vi "IDE_UART_Example.vi"() -> ()   [LabVIEW 2020]
uses:
  Subs/ColorText/Code.xctl
  Subs/Console XCtrl/Console_Xctrl.xctl
  Subs/Server XCtrl/Server.xctl
panel:
  in  "Files 2":bool
  in  "Open Server 2":bool
  in  "Help 2":bool
  in  "Name 2":string="code.py"
  in  "Save 2":bool
  in  "Stop 2":bool
  in  "Pyboard":string(xcontrol)="# UART Control\n#\n# This example shows how to use the serial port on your OpenMV Cam.   P4 (Tx), P5(Rx)\n\nimport utime\nfrom pyb import UART\n\nuart = UART(3, 115200)\n\nwhile(True):\n    if uart.any():\n        uart.read(uart.any())\n    uart.write(\"OpenMV\\r\")\n    utime.sleep(2)\n    \n    \n    "
  in  "Run 2":bool
  in  "Clean 2":bool
  in  "PC Save 2":bool
  in  "PC path 2":path
  in  "Clear 2":bool
  out "REPL 2":string(xcontrol)="\n>>> import time\n>>> from pyb import UART\n>>> uart = UART(3, 19200)\n>>> while(True):\n...     uart.write(\"Hello World!\\r\")\n...     time.sleep(1000)\n...     \n...     \n... \n13\n13\n13\n13\n13\nTraceback (most recent call last):\n  File \"<stdin>\", line 3, in <module>\nKeyboardInterrupt: \n>>> uart.write(\"Hello World!\\r\")\n13\n>>> uart = UART(3, 115200)\n>>> uart.write(\"Hello World!\\r\")\n13\n>>> time.sleep(1)\n>>> time.sleep(1000)\n>>> import utime\n>>> utime.sleep(1)\n>>> import utime\n>>> from pyb import UART\n>>> uart = UART(3, 115200)\n>>> while(True):\n...     if uart.any():\n...         uart.read(uart.any())\n...     uart.write(\"Hello World!\\r\")\n...     utime.sleep(2)\n...     \n...     \n... \n13\n13\n13\nTraceback (most recent call last):\n  File \"<stdin>\", line 5, in <module>\nKeyboardInterrupt: \n>>> import utime\n>>> from pyb import UART\n>>> uart = UART(3, 115200)\n>>> while(True):\n...     if uart.any():\n...         uart.read(uart.any())\n...     uart.write(\"OpenMV\\r\")\n...     utime.sleep(2)\n...     \n...     \n... \n7\nb'SPIKE\\r'\n7\nb'SPIKE\\r'\n7\nb'SPIKE\\r'\n7\nb'SPIKE\\r'\n7\nTraceback (most recent call last):\n  File \"<stdin>\", line 5, in <module>\nKeyboardInterrupt: \n>>> uart.\n__class__       __next__        any             read\nreadinto        readline        write           init\nCTS             IRQ_RXIDLE      RTS             deinit\nirq             readchar        sendbreak       writechar\n>>> uart"
  in  "Server 2":path(xcontrol)=path "/Users/crogers/GitHub/Summer2020/LabVIEWCode/Servers/Damien.vi"
  in  "Clean":bool
  in  "PC Save":bool
  in  "PC path":path
  in  "Files":bool
  in  "Open Server":bool
  in  "Help":bool
  in  "Server":path(xcontrol)=path "/Users/crogers/GitHub/Summer2020/LabVIEWCode/Servers/Jens.vi"
  out "REPL":string(xcontrol)="0], \"\", 0]}{\"m\":0,\"p\":[[0, []], [0, []], [0, []], [0, []], [0, []], [0, []], [-18, -2, 994], [3, 5, 1], [24, 1, 0], \"\", 0]}{\"m\":0,\"p\":[[0, []], [0, []], [0, []], [0, []], [0, []], [0, []], [-19, -3, 994], [3, 6, 1], [24, 1, 0], \"\", 0]}{\"m\":0,\"p\":[[0, []], [0, []], [0, []], [0, []], [0, []], [0, []], [-20, 0, 994], [3, 5, 1], [24, 1, 0], \"\", 0]}Traceback (most recent call last):\n  File \"main.py\", line 8, in <module>\n  File \"lib/hub/flash/hub_runtime.py\", line 1, in start\nKeyboardInterrupt: \nMicroPython v1.11-1139-gf7407e5a0 on 2020-06-19; LEGO Technic Large Hub with STM32F413xx\nType \"help()\" for more information.\n>>> {\"m\":4,\"p\":\"tapped\"}{\"m\":4,\"p\":\"rightside\"}{\"m\":4,\"p\":\"front\"}{\"m\":4,\"p\":\"rightside\"}{\"m\":4,\"p\":\"front\"}{\"m\":4,\"p\":\"tapped\"}\n>>> \n>>> \n>>> {\"m\":4,\"p\":\"tapped\"}\n>>> import hub, utime\n>>> hub.port.B.mode(hub.port.MODE_FULL_DUPLEX)\n>>> utime.sleep(1)\n>>> hub.port.B.baud(115200)\n>>> hub.port.B.write(hello sir!.encode()) \nTraceback (most recent call last):\n  File \"<stdin>\", line 1\nSyntaxError: invalid syntax\n>>> hub.port.B.read(100)\nb''\n>>> \n>>> hub.port.B.write('hello sir!'.encode()) # to write\n10\n>>> hub.port.B.read(100)\nb'hello sir!'\n>>> hub.port.B.read(100)\nb'\\xe0\\xe0\\xe0\\xe0\\xe0\\xe0\\xe0\\xe0\\xe0\\xe0\\xe0\\xe0\\xe0\\xe0\\xe0\\xe0\\xe0\\xe0\\xe0\\xe0\\xe0\\xe0\\xe0\\xe0\\xe0\\xe0\\xe0\\xe0\\xe0\\xe0\\xe0\\xe0\\xe0\\xe0\\xe0\\xe0\\xe0\\xe0\\xe0\\xe0\\xe0\\xe0\\xe0\\xe0\\xe0\\xe0\\xe0\\xe0\\xe0\\xe0\\xe0\\xe0\\xe0\\xe0\\xe0\\xe0\\xe0\\xe0\\xe0\\xe0\\xe0\\xe0\\xe0\\xe0\\xe0\\xe0\\xe0\\xe0\\xe0\\xe0\\xe0\\xe0\\xe0\\xe0\\xe0\\xe0\\xe0\\xe0\\xe0\\xe0\\xe0\\xe0\\xe0\\xe0\\xe0\\xe0\\xe0\\xe0\\xe0\\xe0\\xe0\\xe0\\xe0\\xe0\\xe0\\xe0\\xe0\\xe0\\xe0\\xe0'\n>>> hub.port.B.read(100)\nb'\\xe0\\xe0\\xe0\\xe0\\xe0\\xe0\\xe0\\xe0\\xe0\\xe0\\xe0\\xe0\\xe0\\xe0\\xe0\\xe0\\xe0\\xe0\\xe0\\xe0\\xe0\\xe0\\xe0\\xe0'\n>>> hub.port.B.read(100)\nb''\n>>> hub.port.B.read(100)\nb'\\xe0\\xe0\\xe0\\xe0\\xe0\\xe0\\xe0\\xe0\\xe0\\xe0\\xe0\\xe0\\xe0\\xe0\\xe0\\xe0\\xe0\\xe0\\xe0\\xe0\\xe0\\xe0\\xe0\\xe0\\xe0'\n>>> hub.port.B.read(100)\nb''\n>>> hub.port.B.read(100)\nb'Hello World!\\r'\n>>> \n>>> uart = hub.port.B\n>>> uart.\n__class__       read            write           baud\ncallback        device          info            mode\nmotor           pwm\n>>> uart.read()\nTraceback (most recent call last):\n  File \"<stdin>\", line 1, in <module>\nTypeError: function takes 2 positional arguments but 1 were given\n>>> uart.read(1000)\nb'Hello World!\\rHello World!\\rHello World!\\r'\n>>> import hub, utime\n>>> uart = hub.port.B\n>>> uart.mode(hub.port.MODE_FULL_DUPLEX)\n>>> uart.baud(115200)\n>>> hub.port.B.write('hello sir!'.encode()) \n10\n>>> hub.port.B.read(100)\nb''\n>>> while(True):\n...     uart.read(100)\n...     uart.write(\"SPIKE\\r\")\n...     utime.sleep(2)\n...     \n...     \n... \nb''\n6\nb''\n6\nb'OpenMV\\r'\n6\nb'OpenMV\\r'\n6\nb'OpenMV\\r'\n6\nb'OpenMV\\r'\n6\nTraceback (most recent call last):\n  File \"<stdin>\", line 4, in <module>\nKeyboardInterrupt: \n>>> def gotit():\n...     print(\n>>> {\"m\":4,\"p\":\"tapped\"}"
  in  "Clear":bool
  in  "Save":bool
  in  "Stop":bool
  in  "Run":bool
  in  "Name":string="code.py"
  in  "SPIKE Prime":string(xcontrol)="import hub, utime\n\nuart = hub.port.B\nuart.mode(hub.port.MODE_FULL_DUPLEX)\nuart.baud(115200)\n\nwhile(True):\n    uart.read(100)\n    uart.write(\"SPIKE\\r\")\n    utime.sleep(2)\n    \n    \n    "
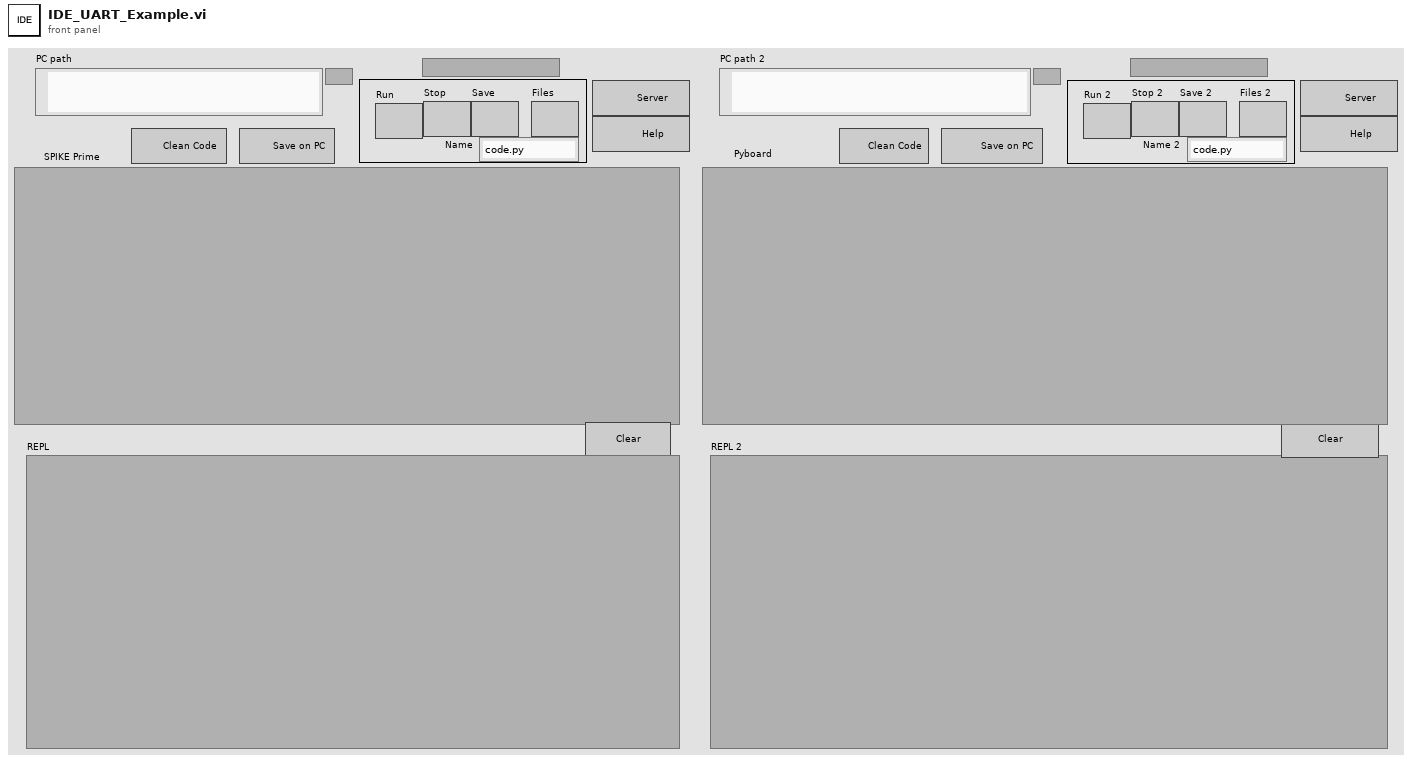
[diagram p1: front panel]
types:
  T1 = cluster{"Quote":u32, "Comment":u32, "Python":u32, "Text":u32, "Triple Quote":u32, "function":u32, "Line numbers":u32, "REPL Err":u32, "REPL Text":u32, "Text Bkgd":u32, "REPL Bkgd":u32}
  T2 = enum8{"Enabled", "Disabled", "Disabled and Grayed Out"}
  T3 = typedef "eventvkey.ctl" = enum16{"ASCII", "Enter", "Return", "Shift", "Ctrl", "Alt", "Cmd", "Opt", "Caps", "NumLock", "Clear", "Break", "Up", "Down", "Left", "Right", "Insert", "Delete", "Home", "End", "PageUp", "PageDown", "Escape", "Help", "Pause", "ScrollLock", "F1", "F2", "F3", "F4", "F5", "F6", "F7", "F8", "F9", "F10", "F11", "F12", "F13", "F14", "F15", "F16", "F17", "F18", "F19", "F20", "F21", "F22", "F23", "F24", "Play", "VolumeUp", "VolumeDown", "Mute", "Two Byte Char"}
  T4 = cluster{"Shift":bool, "Ctrl":bool, "Alt":bool, "Cmd":bool, "Opt":bool}
  T5 = cluster{"Char":i16, "VKey":T3, "PlatMods":cluster{"Shift":bool, "Ctrl":bool, "Alt":bool, "Cmd":bool, "Opt":bool}}
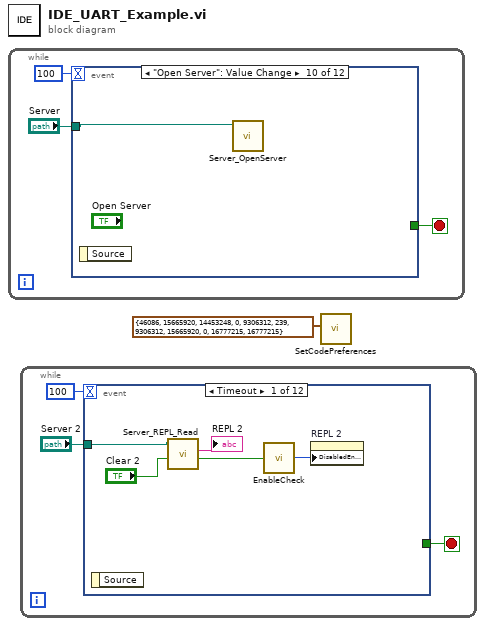
[diagram p0: block diagram]
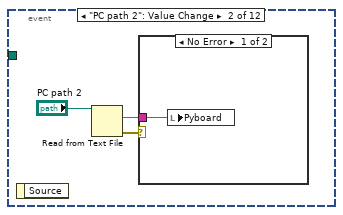
[diagram p2: hidden frame]
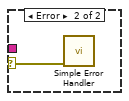
[diagram p3: hidden frame]
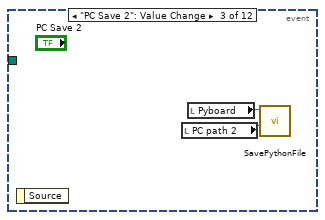
[diagram p4: hidden frame]
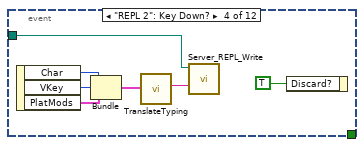
[diagram p5: hidden frame]
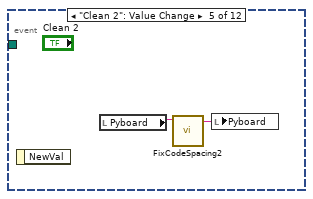
[diagram p6: hidden frame]
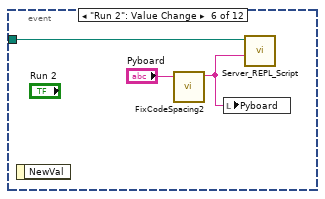
[diagram p7: hidden frame]
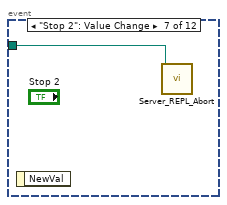
[diagram p8: hidden frame]
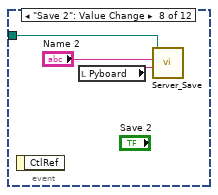
[diagram p9: hidden frame]
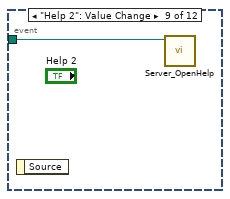
[diagram p10: hidden frame]
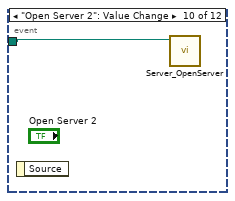
[diagram p11: hidden frame]
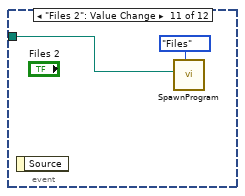
[diagram p12: hidden frame]
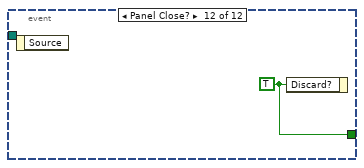
[diagram p13: hidden frame]
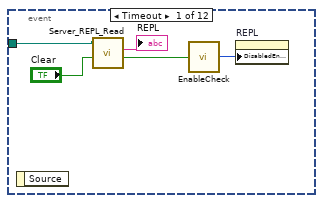
[diagram p14: hidden frame]
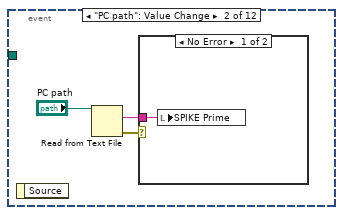
[diagram p15: hidden frame]
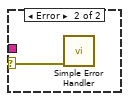
[diagram p16: hidden frame]
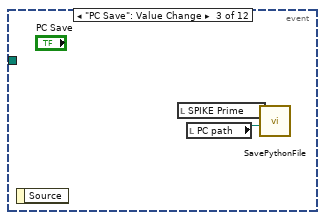
[diagram p17: hidden frame]
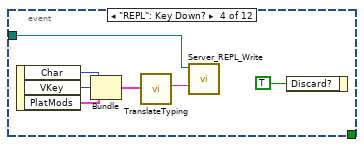
[diagram p18: hidden frame]
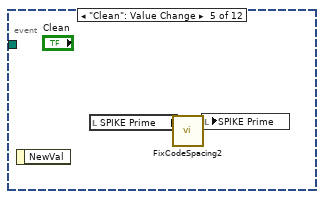
[diagram p19: hidden frame]
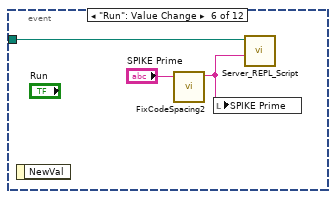
[diagram p20: hidden frame]
diagram:
  n1 = while {
    stop <- w3 stop-if-true
    n2 = event shown="[9] \"Open Server\": Value Change" {
      selector: _ -> [_ _ _ _ _ _ _ _ _ _ _ _]
      dyn-events: _ -> [_ _ _ _ _ _ _ _ _ _ _ _]
      timeout: 100 -> [_ _ _ _ _ _ _ _ _ _ _ _]
      tunnel: [_ _ _ _ _ _ _ _ _ _ _ w37] -> w3
      tunnel: "Server" -> [w7 _ _ w17 _ w27 w29 w30 w33 w34 w36 _]
      event Timeout {
        n3 = event-data() -> ()  [unwired: 1 in, 1 out]
        n4 = call "Server_REPL_Read.vi"("Clear"="Clear", "Server"=w7) -> ("Running?"=w8:bool, "REPL"=→"REPL":string)  [unwired: 7 in, 1 out]
        n5 = call "EnableCheck.vi"("Enable?"=w8) -> ("Enum"=w9:T2)
        n6 = property on="REPL" class="Console_Xctrl (strict)"("DisabledEnum"=w9) -> ()  [unwired: 2 in, 2 out]
      }
      event "PC path": Value Change {
        n7 = event-data() -> ()  [unwired: 1 in, 1 out]
        n8 = Read from Text File(file (use dialog)="PC path") -> (text=w11:string, error out=w12:errorcluster)  [unwired: 3 in, 2 out]
        n9 = case shown="No Error" w12 {
          selector: w12 -> [_ w14]
          tunnel: w11 -> [w13 _]
          frame No Error {
            n10 = local write "SPIKE Prime"(w13) -> ()
          }
          frame Error {
            n11 = call <vilib>:"Simple Error Handler.vi"("error in (no error)"=w14) -> ()  [unwired: 4 in, 5 out]
          }
        }
      }
      event "PC Save": Value Change {
        n12 = event-data() -> ()  [unwired: 1 in, 1 out]
        n13 = local read "SPIKE Prime"() -> (w16:string)
        n14 = local read "PC path"() -> (w15:path)
        n15 = call "SavePythonFile.vi"("path"=w15, "Code"=w16) -> ()  [unwired: 10 in]
      }
      event "REPL": Key Down? {
        n16 = event-data() -> ("Char"=w22:i16, "VKey"=w21:T3, "PlatMods"=w19:T4)  [unwired: 1 in]
        n17 = Bundle("Char"=w22, "VKey"=w21, "PlatMods"=w19) -> (w23:T5)  [unwired: 1 in]
        n18 = call "TranslateTyping.vi"("Cluster"=w23) -> ("key"=w18:string)  [unwired: 10 in]
        n19 = call "Server_REPL_Write.vi"("Code"=w18, "Server"=w17) -> ()  [unwired: 9 in, 1 out]
        n20 = event-data("Discard?"=TRUE) -> ()  [unwired: 1 in, 1 out]
      }
      event "Clean": Value Change {
        n21 = event-data() -> ()  [unwired: 1 in, 1 out]
        n22 = local read "SPIKE Prime"() -> (w24:string)
        n23 = call "FixCodeSpacing2.vi"("Code"=w24) -> ("Cleaned"=w25:string)  [unwired: 10 in]
        n24 = local write "SPIKE Prime"(w25) -> ()
      }
      event "Run": Value Change {
        n25 = event-data() -> ()  [unwired: 1 in, 1 out]
        n26 = call "FixCodeSpacing2.vi"("Code"="SPIKE Prime") -> ("Cleaned"=w26:string)  [unwired: 10 in]
        n27 = local write "SPIKE Prime"(w26) -> ()
        n28 = call "Server_REPL_Script.vi"("Code"=w26, "Server"=w27) -> ()  [unwired: 9 in, 1 out]
      }
      event "Stop": Value Change {
        n29 = event-data() -> ()  [unwired: 1 in, 1 out]
        n30 = call "Server_REPL_Abort.vi"("Server"=w29) -> ()  [unwired: 10 in, 1 out]
      }
      event "Save": Value Change {
        n31 = event-data() -> ()  [unwired: 1 in, 1 out]
        n32 = local read "SPIKE Prime"() -> (w32:string)
        n33 = call "Server_Save.vi"("Code"=w32, "Name"="Name", "Server"=w30) -> ()  [unwired: 8 in, 1 out]
      }
      event "Help": Value Change {
        n34 = event-data() -> ()  [unwired: 1 in, 1 out]
        n35 = call "Server_OpenHelp.vi"("Server"=w33) -> ()  [unwired: 10 in, 1 out]
      }
      event "Open Server": Value Change {
        n36 = event-data() -> ()  [unwired: 1 in, 1 out]
        n37 = call "Server_OpenServer.vi"("Server"=w34) -> ()  [unwired: 10 in, 1 out]
      }
      event "Files": Value Change {
        n38 = event-data() -> ()  [unwired: 1 in, 1 out]
        n39 = call "SpawnProgram.vi"("Server"=w36, "Dialog"=enum16{"Help", "Files"}."Files") -> ()  [unwired: 10 in]
      }
      event Panel Close? {
        w37 = TRUE ("Discard?")
        n40 = event-data() -> ()  [unwired: 1 in, 1 out]
        n41 = event-data("Discard?"=w37) -> ()  [unwired: 1 in, 1 out]
      }
    }
  }
  n42 = while {
    stop <- w39 stop-if-true
    n43 = event shown="[0] Timeout" {
      selector: _ -> [_ _ _ _ _ _ _ _ _ _ _ _]
      dyn-events: _ -> [_ _ _ _ _ _ _ _ _ _ _ _]
      timeout: 100 -> [_ _ _ _ _ _ _ _ _ _ _ _]
      tunnel: [_ _ _ _ _ _ _ _ _ _ _ w73] -> w39
      tunnel: "Server 2" -> [w43 _ _ w53 _ w63 w65 w66 w69 w70 w72 _]
      event Timeout {
        n44 = event-data() -> ()  [unwired: 1 in, 1 out]
        n45 = call "Server_REPL_Read.vi"("Clear"="Clear 2", "Server"=w43) -> ("Running?"=w44:bool, "REPL"=→"REPL 2":string)  [unwired: 7 in, 1 out]
        n46 = call "EnableCheck.vi"("Enable?"=w44) -> ("Enum"=w45:T2)
        n47 = property on="REPL 2" class="Console_Xctrl (strict)"("DisabledEnum"=w45) -> ()  [unwired: 2 in, 2 out]
      }
      event "PC path 2": Value Change {
        n48 = event-data() -> ()  [unwired: 1 in, 1 out]
        n49 = Read from Text File(file (use dialog)="PC path 2") -> (text=w47:string, error out=w48:errorcluster)  [unwired: 3 in, 2 out]
        n50 = case shown="No Error" w48 {
          selector: w48 -> [_ w50]
          tunnel: w47 -> [w49 _]
          frame No Error {
            n51 = local write "Pyboard"(w49) -> ()
          }
          frame Error {
            n52 = call <vilib>:"Simple Error Handler.vi"("error in (no error)"=w50) -> ()  [unwired: 4 in, 5 out]
          }
        }
      }
      event "PC Save 2": Value Change {
        n53 = event-data() -> ()  [unwired: 1 in, 1 out]
        n54 = local read "PC path 2"() -> (w51:path)
        n55 = local read "Pyboard"() -> (w52:string)
        n56 = call "SavePythonFile.vi"("path"=w51, "Code"=w52) -> ()  [unwired: 10 in]
      }
      event "REPL 2": Key Down? {
        n57 = event-data() -> ("Char"=w58:i16, "VKey"=w57:T3, "PlatMods"=w55:T4)  [unwired: 1 in]
        n58 = Bundle("Char"=w58, "VKey"=w57, "PlatMods"=w55) -> (w59:T5)  [unwired: 1 in]
        n59 = call "TranslateTyping.vi"("Cluster"=w59) -> ("key"=w54:string)  [unwired: 10 in]
        n60 = call "Server_REPL_Write.vi"("Code"=w54, "Server"=w53) -> ()  [unwired: 9 in, 1 out]
        n61 = event-data("Discard?"=TRUE) -> ()  [unwired: 1 in, 1 out]
      }
      event "Clean 2": Value Change {
        n62 = event-data() -> ()  [unwired: 1 in, 1 out]
        n63 = local read "Pyboard"() -> (w60:string)
        n64 = call "FixCodeSpacing2.vi"("Code"=w60) -> ("Cleaned"=w61:string)  [unwired: 10 in]
        n65 = local write "Pyboard"(w61) -> ()
      }
      event "Run 2": Value Change {
        n66 = event-data() -> ()  [unwired: 1 in, 1 out]
        n67 = call "FixCodeSpacing2.vi"("Code"="Pyboard") -> ("Cleaned"=w62:string)  [unwired: 10 in]
        n68 = local write "Pyboard"(w62) -> ()
        n69 = call "Server_REPL_Script.vi"("Code"=w62, "Server"=w63) -> ()  [unwired: 9 in, 1 out]
      }
      event "Stop 2": Value Change {
        n70 = event-data() -> ()  [unwired: 1 in, 1 out]
        n71 = call "Server_REPL_Abort.vi"("Server"=w65) -> ()  [unwired: 10 in, 1 out]
      }
      event "Save 2": Value Change {
        n72 = event-data() -> ()  [unwired: 1 in, 1 out]
        n73 = local read "Pyboard"() -> (w68:string)
        n74 = call "Server_Save.vi"("Code"=w68, "Name"="Name 2", "Server"=w66) -> ()  [unwired: 8 in, 1 out]
      }
      event "Help 2": Value Change {
        n75 = event-data() -> ()  [unwired: 1 in, 1 out]
        n76 = call "Server_OpenHelp.vi"("Server"=w69) -> ()  [unwired: 10 in, 1 out]
      }
      event "Open Server 2": Value Change {
        n77 = event-data() -> ()  [unwired: 1 in, 1 out]
        n78 = call "Server_OpenServer.vi"("Server"=w70) -> ()  [unwired: 10 in, 1 out]
      }
      event "Files 2": Value Change {
        n79 = event-data() -> ()  [unwired: 1 in, 1 out]
        n80 = call "SpawnProgram.vi"("Server"=w72, "Dialog"=enum16{"Help", "Files"}."Files") -> ()  [unwired: 10 in]
      }
      event Panel Close? {
        w73 = TRUE ("Discard?")
        n81 = event-data() -> ()  [unwired: 1 in, 1 out]
        n82 = event-data("Discard?"=w73) -> ()  [unwired: 1 in, 1 out]
      }
    }
  }
  n83 = call "SetCodePreferences.vi"("Color choices"=T1 {"Quote"=46086, "Comment"=15665920, "Python"=14453248, "Text"=0, "Triple Quote"=9306312, "function"=239, "Line numbers"=9306312, "REPL Err"=15665920, "REPL Text"=0, "Text Bkgd"=16777215, "REPL Bkgd"=16777215}) -> ()  [unwired: 11 in]
